vi "Measure Sound from Digital Mic - PDM and I2S.vi"() -> ()   [LabVIEW 2022 SP3]
doc: "This example performs a continuous acquisition of PCM data. At the same time, the GPIO lines are used for digital input and digital output."
uses:
  source/shared/controls/input type.ctl
  <vilib>/PDM Acquisition Toolkit/host/Classes/Tasks/PDM Tasks/Controls/Acquisition Mode.ctl
  <vilib>/PDM Acquisition Toolkit/shared/controls/clock mode.ctl
  <vilib>/addons/_NISVFA/_Shared subVIs/Common/SVL Set dB Reference (1 Ch).vi
  <vilib>/addons/Sound and Vibration/svt_Level/SVL AC & DC Level (Time) (1 Ch).vi
  <vilib>/addons/_NISVFA/_Shared subVIs/Common/SVL Set dB Reference (variant).vi
  <vilib>/addons/_NISVFA/_Shared subVIs/Common/svc_Get SV Channel Info.vi
  <vilib>/Analysis/baseanly.llb/Mean.vi
  <vilib>/Analysis/baseanly.llb/Mean (DBL).vi
  <vilib>/addons/_NISVFA/_Shared subVIs/Windowing/svfa_Scaled Time Domain Window (Array).vi
  <vilib>/addons/_NISVFA/_Shared subVIs/Common/svc_Unit Label to Engineering Units.vi
  <vilib>/addons/_NISVFA/_Shared subVIs/Common/svc_Engineering Units to Unit Label.vi
  <vilib>/addons/_NISVFA/_Spectrum Processing/subVIs/svfa_Spectrum Info Window to windowTd Type Def.vi
  <vilib>/Analysis/4window.llb/Force Window.vi
  <vilib>/Analysis/4window.llb/Force Window (DBL).vi
  <vilib>/Analysis/4window.llb/Exponential Window.vi
  <vilib>/Analysis/4window.llb/Exponential Window (DBL).vi
  <vilib>/PDM Acquisition Toolkit/host/API/Public/Create Tasks/Create PCM Input Task.vi
  <vilib>/PDM Acquisition Toolkit/host/API/Public/Configure/Timing/Configure Timing - PCM Input Master.vi
  <vilib>/PDM Acquisition Toolkit/host/API/Public/Configure/PDM Channel/Configure Microphone Sensitivity DBFS - PCM Input Task.vi
  <vilib>/PDM Acquisition Toolkit/host/API/Public/Start/Start PCM Input Task.vi
  source/shared/task conversion/From PCM task.vi
  <vilib>/PDM Acquisition Toolkit/host/API/Public/Create Tasks/Create PDM Input Task.vi
  <vilib>/PDM Acquisition Toolkit/host/API/Public/Configure/Timing/Configure Timing - PDM Input.vi
  <vilib>/PDM Acquisition Toolkit/host/API/Public/Configure/PDM Channel/Configure Microphone Sensitivity DBFS.vi
  source/shared/task conversion/From PDM task.vi
  source/shared/task conversion/To PCM task.vi
  <vilib>/PDM Acquisition Toolkit/host/API/Public/Read/Read PCM Input Waveform.vi
  source/shared/task conversion/To PDM task.vi
  <vilib>/PDM Acquisition Toolkit/host/API/Public/Read/Read PCM Waveform.vi
  <vilib>/addons/_NISVFA/_Shared subVIs/Common/svc_Caller VI Returned in Error Source.vi
  <vilib>/addons/_NISVFA/_Shared subVIs/Common/svc_Get Window Info.vi
  <vilib>/Analysis/0measdsp.llb/Scaled Time Domain Window.vi
  <vilib>/Analysis/0measdsp.llb/Scaled Time Domain Window (DBL).vi
  <vilib>/Utility/error.llb/Error Cluster From Error Code.vi
  <vilib>/Analysis/baseanly.llb/Std Deviation and Variance.vi
  <vilib>/addons/Sound and Vibration/svt_Weighting/SVT Weighting Filter (1 Ch).vi
  <vilib>/addons/Sound and Vibration/svt_Level/SVL Leq Sound Level (1 Ch).vi
  <vilib>/PDM Acquisition Toolkit/host/API/Public/Clear/Clear PDM Input Task.vi
  <vilib>/PDM Acquisition Toolkit/host/API/Public/Stop/Stop PCM Input Task.vi
  <vilib>/PDM Acquisition Toolkit/host/API/Public/Clear/Clear PCM Input Task.vi
  <vilib>/PDM Acquisition Toolkit/host/API/PDM Acquisition Toolkit.lvlib
  <vilib>/PDM Acquisition Toolkit/host/Classes/Tasks/PDM Tasks/PDM Task.lvclass
  <vilib>/PDM Acquisition Toolkit/shared/PDM Shared.lvlib
  <vilib>/addons/Sound and Vibration/svt_Weighting/SoundVib_ABCWeighting.lvlib
  <vilib>/addons/Sound and Vibration/svt_Level/SoundVib_SoundLevel.lvlib
  source/shared/input configuration file/input cfg file.lvlib
  source/shared/input configuration file/digital serial/digital serial input cfg file.lvlib
  source/shared/input configuration file/PDM/PDM input cfg file.lvlib
  source/shared/task conversion/DAAG task conversion.lvlib
panel:
  out "input cfg JSON":string
  out "input type":T1 caption="master clock source"
  in  "File Path":path
  out "Leq sound level [dB EU]":dbl=63.21387111345029 format="%.2f"
  in  "weighting":u16(ring) items=["Linear", "A-weighting", "B-weighting", "C-weighting"]
  out "Error Out":errorcluster
  out "Waveform Graph":waveform(dbl)(graph)={"t0"=timestamp(0 s since 1904-01-01), "dt"=2.0833333385932442e-05, "Y"=[], "attributes"=variant("NI_ChannelName"=variant(string "PDMI0L"), "NI_dBReference"=variant(dbl 2e-05))}
  in  "Number of Samples":i32=12000
  in  "PDM Channels":string="PXI1Slot5\\PDMi 0"
  in  "Microphone Sensitivity (dBFS)":dbl=-26.0 format="%#_13g"
  in  "Stop":bool
  # "PDM Input"
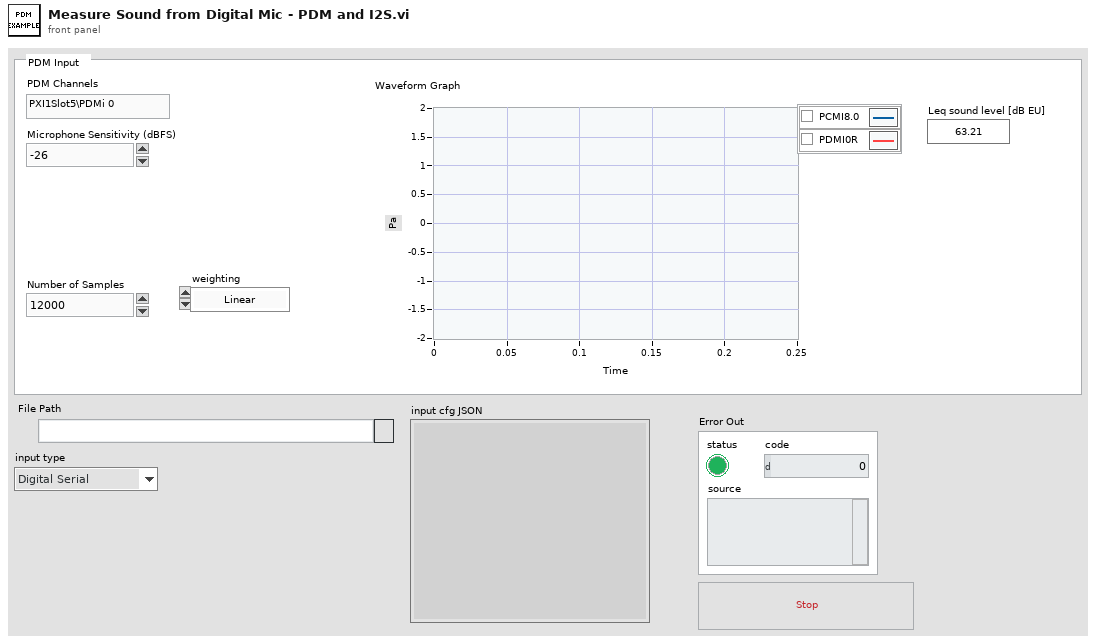
[diagram p1: front panel]
types:
  T1 = typedef "input type.ctl" = enum32{"Digital Serial", "PDM"}
  T2 = typedef "PDM Shared.lvlib/clock mode.ctl" = enum16{"divided clock", "DDS"}
  T3 = typedef "PDM Acquisition Class Library.lvlib/PDM Task.lvclass/Acquisition Mode.ctl" = enum16{"Finite", "Continuous"}
  T4 = typedef "digital serial input settings.ctl" = cluster{"number of channels":u32, "data justification":T5, "endianness":T6, "channel length":u32, "bit depth":u32, "frame clock rate":dbl, "bit clock edge sync":T7, "master clock source":T8, "master clock rate":dbl, "Logic Level":T9, "frame sync edge for channel 0":T7, "Channel 0 Offset":u32}
  T5 = typedef "PDM Shared.lvlib/PCM Data Justification.ctl" = enum16{"Left Justified", "Right Justified"}
  T6 = typedef "PDM Shared.lvlib/PCM Bit Endianness.ctl" = enum16{"MSB First", "LSB First"}
  T7 = typedef "PDM Shared.lvlib/Digital Edge.ctl" = enum8{"Rising", "Falling"}
  T8 = typedef "master clock source.ctl" = enum32{"Internal", "External"}
  T9 = typedef "PDM Acquisition Class Library.lvlib/DecoderSession.lvclass/Logic Levels.ctl" = enum16{"3.3 V", "1.8 V", "1.2 V"}
  T10 = typedef "PDM Shared.lvlib/PCM Frame Sync Control.ctl" = cluster{"Frame Length":u16, "Frame Sync Pulse Width":u16, "Bit Clock Edge  Sync":T7}
  T11 = typedef "PDM Shared.lvlib/PCM Data Format Configuration.ctl" = cluster{"Frame Sync Edge for Channel 0":T7, "Channel Count Per Frame":u8, "Channel Length":u16, "Bit Depth":u8, "Channel 0 Offset":u16, "Endianness":T6, "Data Justification":T5}
  T12 = typedef "PDM Acquisition Class Library.lvlib/PCM Input Task.lvclass/DVR PCM Input Task.ctl" = refnum<data-value>
  T13 = typedef "PDM input settings.ctl" = cluster{"PDM clock rate":dbl, "decimation factor":T14, "bit clock direction":T15, "logic level":T9}
  T14 = typedef "PDM Shared.lvlib/decimation order.ctl" = u16
  T15 = typedef "bit clock direction.ctl" = enum32{"In", "Out"}
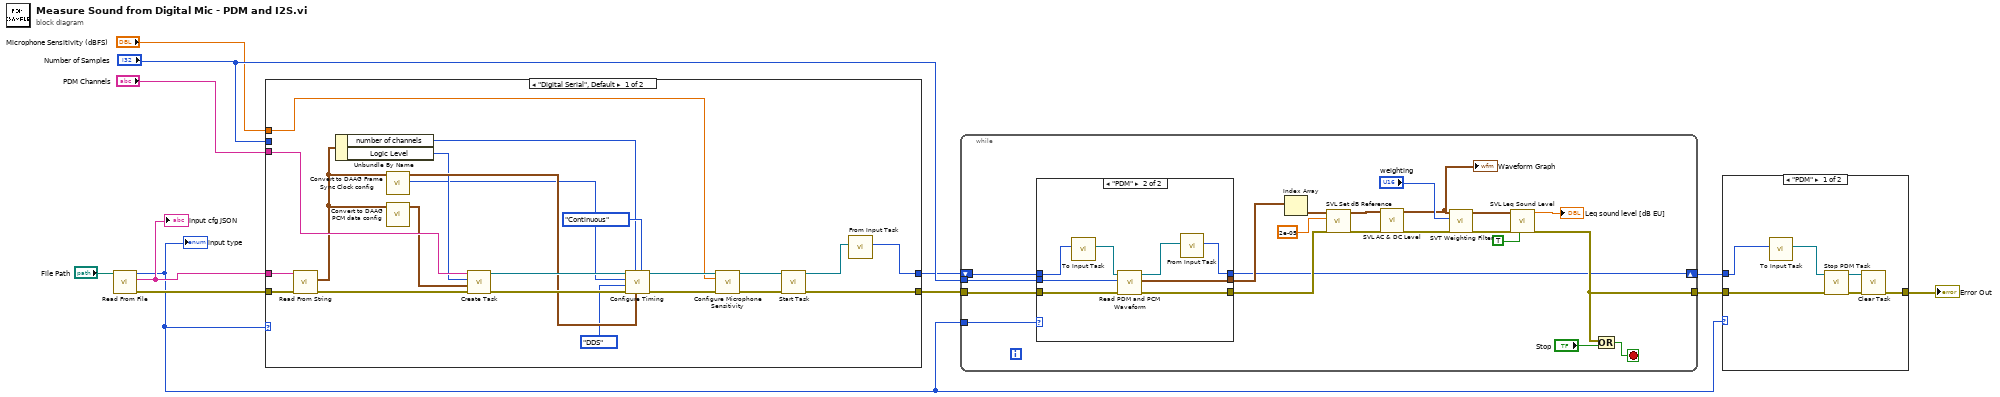
[diagram p0: block diagram]
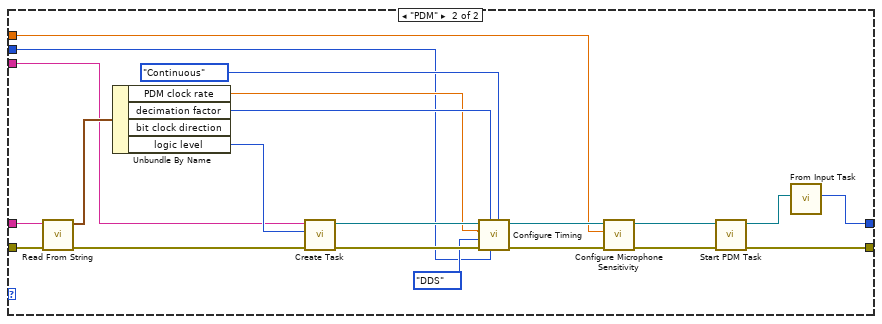
[diagram p2: hidden frame]
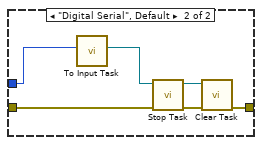
[diagram p3: hidden frame]
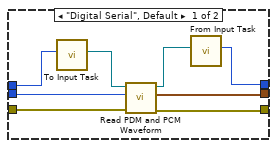
[diagram p4: hidden frame]
diagram:
  n1 = call "Read From File.vi"("file path"="File Path") -> ("error out"=w10:errorcluster, "input cfg JSON"=w9:string, "input type"=w1:T1)  [unwired: 7 in, 1 out]
  "input type" <- w1
  "input cfg JSON" <- w9
  n2 = case shown="\"Digital Serial\", Default" w1 {
    tunnel: w10 -> [w34 w55]
    tunnel: w9 -> [w33 w54]
    tunnel: "Number of Samples" -> [_ w43]
    tunnel: "PDM Channels" -> [w24 w44]
    tunnel: [w25 w38] -> w4
    tunnel: "Microphone Sensitivity (dBFS)" -> [w16 w37]
    tunnel: [w13 w35] -> w3
    frame "Digital Serial", Default {
      n3 = call "Read From String.vi"("error in (no error)"=w34, "JSON string"=w33) -> ("error out"=w32:errorcluster, "digital serial input settings"=w23:T4)  [unwired: 8 in]
      n4 = Unbundle By Name(w23) -> ("number of channels"=w19:u32, "Logic Level"=w18:T9)
      n5 = call "Convert to DAAG Frame Sync Clock config.vi"("digital serial input settings"=w23) -> ("Bit Clock rate"=w15:u32, "Frame Sync Clock Control"=w21:T10)  [unwired: 9 in]
      n6 = call "Convert to DAAG PCM data config.vi"("digital serial input settings"=w23) -> ("PCM data configuration"=w22:T11)  [unwired: 10 in]
      n7 = call-poly <vilib>:"Create Task.vi"("error in"=w32, "PCM data configuration"=w22, "logic level"=w18, "channel list"=w24) -> ("error out"=w30:errorcluster, "PCM input task out"=w31:T12)  [unwired: 6 in]
      n8 = call-poly <vilib>:"Configure Timing.vi"("acquisition mode"=Acquisition_Mode."Continuous", "Frame Sync Clock Control"=w21, "number of words per channel"=w19, "error in"=w30, "clock mode"=clock_mode."DDS", "Bit Clock rate"=w15, "PCM input task in"=w31) -> ("error out"=w27:errorcluster, "PCM input task out"=w28:T12)  [unwired: 2 in, 1 out]
      n9 = call-poly <vilib>:"Configure Microphone Sensitivity.vi"("error in"=w27, "microphone sensitivity (dBFS)"=w16, "PCM input task in"=w28) -> ("error out"=w29:errorcluster, "PCM input task out"=w26:T12)  [unwired: 7 in]
      n10 = call-poly <vilib>:"Start Task.vi"("error in"=w29, "PCM input task in"=w26) -> ("error out"=w25:errorcluster, "PCM input task out"=w14:T12)  [unwired: 8 in]
      n11 = call-poly "From Input Task.vi"("PCM input task"=w14) -> ("task"=w13:u64)  [unwired: 10 in]
    }
    frame "PDM" {
      n12 = call "Read From String.vi"("error in (no error)"=w55, "JSON string"=w54) -> ("error out"=w52:errorcluster, "input settings"=w53:T13)  [unwired: 8 in]
      n13 = Unbundle By Name(w53) -> ("PDM clock rate"=w46:dbl, "decimation factor"=w47:T14, "logic level"=w49:T9)  [unwired: 1 out]
      n14 = call-poly <vilib>:"Create Task.vi"("error in"=w52, "logic level"=w49, "channel list"=w44) -> ("error out"=w50:errorcluster, "PDM input task out"=w51:refnum<data-value>)  [unwired: 7 in]
      n15 = call-poly <vilib>:"Configure Timing.vi"("acquisition mode"=Acquisition_Mode."Continuous", "number of PCM samples"=w43, "decimation factor"=w47, "error in"=w50, "clock mode"=clock_mode."DDS", "PDM clock rate"=w46, "PDM input task in"=w51) -> ("error out"=w41:errorcluster, "PDM input task out"=w42:refnum<data-value>)  [unwired: 1 in, 2 out]
      n16 = call-poly <vilib>:"Configure Microphone Sensitivity.vi"("error in"=w41, "microphone sensitivity (dBFS)"=w37, "PDM input task in"=w42) -> ("error out"=w39:errorcluster, "PDM input task out"=w40:refnum<data-value>)  [unwired: 7 in]
      n17 = call <vilib>:"Start PDM Task.vi"("error in"=w39, "PDM input task in"=w40) -> ("error out"=w38:errorcluster, "PDM input task out"=w36:refnum<data-value>)  [unwired: 8 in]
      n18 = call-poly "From Input Task.vi"("PDM input task"=w36) -> ("task"=w35:u64)  [unwired: 10 in]
    }
  }
  n19 = while {
    tunnel: w4 -> [w76]
    tunnel: "Number of Samples" -> [w75]
    shift-right: [w56] -> w2
    shift-left: w3 -> [w58]
    tunnel: [w59] -> w11
    tunnel: w1 -> [w57]
    stop <- w74 stop-if-true
    n20 = case shown="\"PDM\"" w57 {
      tunnel: w76 -> [w84 w92]
      tunnel: w75 -> [w83 w91]
      tunnel: [w81 w90] -> w66
      tunnel: [w82 w89] -> w64
      tunnel: w58 -> [w80 w88]
      tunnel: [w77 w85] -> w56
      frame "Digital Serial", Default {
        n21 = call-poly "To Input Task.vi"("task"=w80) -> ("PCM task"=w79:T12)  [unwired: 10 in]
        n22 = call-poly <vilib>:"Read PDM and PCM Waveform.vi"("error in"=w84, "words per channel"=w83, "PCM input task In"=w79) -> ("error out"=w81:errorcluster, "PCM waveforms"=w82:waveform(dbl)[], "PCM input task out"=w78:T12)  [unwired: 3 in, 3 out]
        n23 = call-poly "From Input Task.vi"("PCM input task"=w78) -> ("task"=w77:u64)  [unwired: 10 in]
      }
      frame "PDM" {
        n24 = call-poly "To Input Task.vi"("task"=w88) -> ("PDM task"=w87:refnum<data-value>)  [unwired: 10 in]
        n25 = call-poly <vilib>:"Read PDM and PCM Waveform.vi"("error in"=w92, "samples per channel"=w91, "PDM input task in"=w87) -> ("error out"=w90:errorcluster, "PCM waveforms"=w89:waveform(dbl)[], "PDM input task out"=w86:refnum<data-value>)  [unwired: 5 in, 1 out]
        n26 = call-poly "From Input Task.vi"("PDM input task"=w86) -> ("task"=w85:u64)  [unwired: 10 in]
      }
    }
    n27 = Index Array(array=w64) -> (element=w67:waveform(dbl))  [unwired: 1 in]
    n28 = call-poly <vilib>:"SVL Set dB Reference.vi"("error in (no error)"=w66, "dB reference [EU]"=2e-05, "scaled signal in [EU]"=w67) -> ("error out"=w60:errorcluster, "scaled signal out [EU]"=w63:waveform(dbl))  [unwired: 7 in]
    n29 = call-poly <vilib>:"SVL AC & DC Level.vi"("scaled signal [EU]"=w63, "error in (no error)"=w60) -> ("AC signal [EU]"=w62:waveform(dbl), "error out"=w61:errorcluster)  [unwired: 12 in, 4 out]
    "Waveform Graph" <- w62
    n30 = call-poly <vilib>:"SVT Weighting Filter.vi"("error in (no error)"=w61, "weighting"="weighting", "scaled signal [EU]"=w62) -> ("error out"=w71:errorcluster, "weighted signal [EU]"=w68:waveform(dbl))  [unwired: 6 in]
    n31 = call-poly <vilib>:"SVL Leq Sound Level.vi"("restart averaging (F)"=TRUE, "error in (no error)"=w71, "scaled signal [EU]"=w68) -> ("error out"=w59:errorcluster, "Leq sound level [dB EU]"=→"Leq sound level [dB EU]":dbl)  [unwired: 6 in, 1 out]
    n32 = Or(x=w59, y="Stop") -> (x .or. y?=w74:bool)
  }
  n33 = case shown="\"PDM\"" w1 {
    tunnel: [w96 w101] -> w12
    tunnel: w11 -> [w95 w102]
    tunnel: w2 -> [w94 w100]
    frame "PDM" {
      n34 = call-poly "To Input Task.vi"("task"=w94) -> ("PDM task"=w93:refnum<data-value>)  [unwired: 10 in]
      n35 = call <vilib>:"Stop PDM Task.vi"("error in"=w95, "PDM input task in"=w93) -> ("error out"=w97:errorcluster, "PDM input task out"=w98:refnum<data-value>)  [unwired: 8 in]
      n36 = call-poly <vilib>:"Clear Task.vi"("error in"=w97, "PDM input task in"=w98) -> ("error out"=w96:errorcluster)  [unwired: 9 in]
    }
    frame "Digital Serial", Default {
      n37 = call-poly "To Input Task.vi"("task"=w100) -> ("PCM task"=w99:T12)  [unwired: 10 in]
      n38 = call-poly <vilib>:"Stop Task.vi"("error in"=w102, "PCM input task In"=w99) -> ("error out"=w103:errorcluster, "PCM input task out"=w104:T12)  [unwired: 8 in]
      n39 = call-poly <vilib>:"Clear Task.vi"("error in"=w103, "PCM input task in"=w104) -> ("error out"=w101:errorcluster)  [unwired: 9 in]
    }
  }
  "Error Out" <- w12
